vi "購買土地.vi"() -> (1 "確定 2":bool)   [LabVIEW 2014]
panel:
  in  "取消":bool
  in  "確定":bool
  out "Color Box":u32(colorbox)=16768479
  # "要購買土地嗎？"
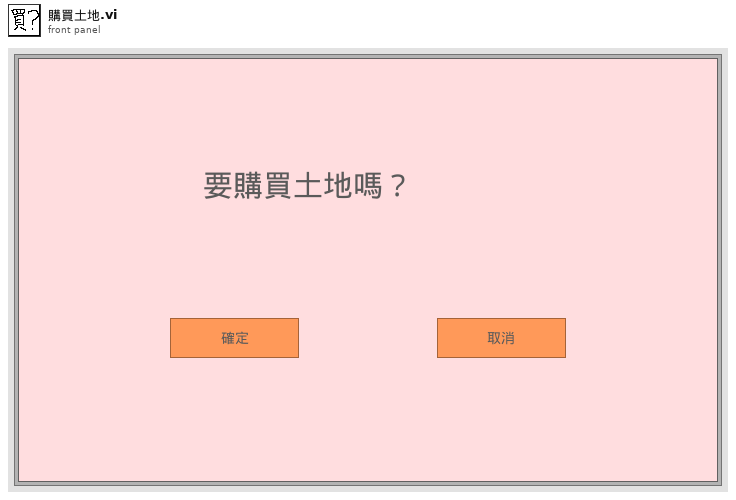
[diagram p1: front panel]
types:
  T1 = enum8{"Enabled", "Disabled", "Disabled and Grayed Out"}
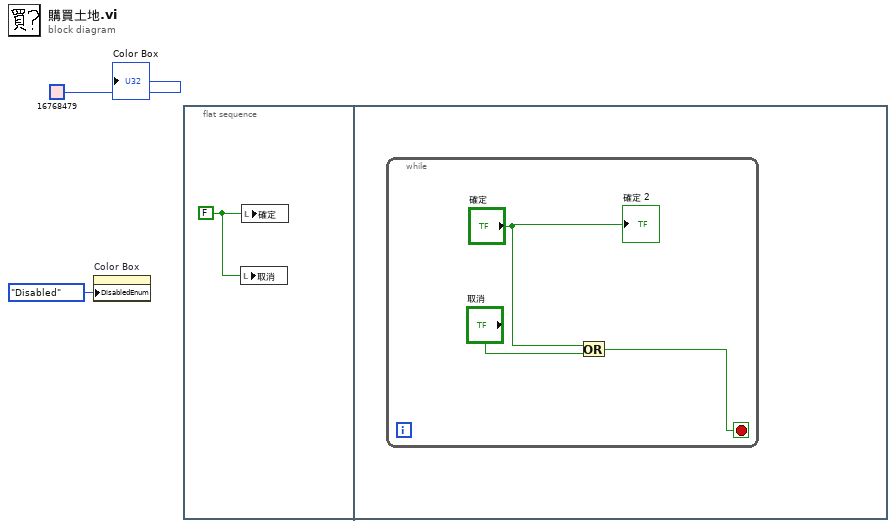
[diagram p0: block diagram]
diagram:
  n1 = property on="Color Box" class="ColBox"("DisabledEnum"=T1."Disabled" ("Disabled")) -> ()  [unwired: 2 in, 2 out]
  n2 = flat-sequence {
    frame #0 {
      w3 = FALSE ("確定")
      n3 = local write "取消"(w3) -> ()
      n4 = local write "確定"(w3) -> ()
    }
    frame #1 {
      n5 = while {
        stop <- w4 stop-if-true
        n6 = Or(x="確定", y="取消") -> (x .or. y?=w4:bool)
        "確定 2" <- "確定"
      }
    }
  }
  "Color Box" <- u32 16768479 ("Color Box")
